vi "Byte to BCD.vi"(11 "U8":u8 format="%08x") -> (2 "low nibble":u8 format="%d\n%04b", 3 "hi nibble":u8 format="%d\n%04b")   [LabVIEW 2015, in "PAS.lvclass"]
uses:
  PAS.lvclass
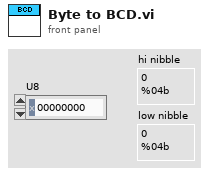
[diagram p1: front panel]
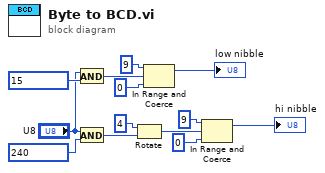
[diagram p0: block diagram]
diagram:
  n1 = And(x="U8", y=u8 15) -> (x .and. y?=w8:u8)
  n2 = And(x="U8", y=u8 240) -> (x .and. y?=w10:u8)
  n3 = Rotate(1:w10, 2:u8 4 ("x")) -> (0:w3:u8)
  n4 = In Range and Coerce(upper limit=u8 9, x=w8, lower limit=u8 0) -> (coerced(x)=→"low nibble":u8)  [unwired: 1 out]
  n5 = In Range and Coerce(upper limit=u8 9, x=w3, lower limit=u8 0) -> (coerced(x)=→"hi nibble":u8)  [unwired: 1 out]
